vi "ELVIS III v1.0 Build MUX Configuration DIO.vi"(11 "DIO Channel List":T4) -> (1 "Configuration Bitmask Array":bool[][](array[boolean]), 2 "Configration Bitcode Array":bool[][](array[boolean]), 3 "Channel Reservation List":T1)   [LabVIEW 2021]
uses:
  <vilib>/myRIO/Common/Instrument Driver Framework/myRIO v1.0/DIO/typedefs/DIO Channels List.ctl
  <vilib>/myRIO/Common/Instrument Driver Framework/myRIO v1.0/DIO/typedefs/DIO Channels Enum.ctl
  <vilib>/myRIO/Common/Instrument Driver Framework/ELVIS III v1.0/Resource Manager/typedefs/ELVIS III v1.0 Channel Reservation List.ctl
  <vilib>/myRIO/Common/Instrument Driver Framework/ELVIS III v1.0/Resource Manager/typedefs/ELVIS III v1.0 Channel Reservation Info.ctl
  <vilib>/myRIO/Common/Instrument Driver Framework/ELVIS III v1.0/Resource Manager/typedefs/ELVIS III v1.0 Connector List.ctl
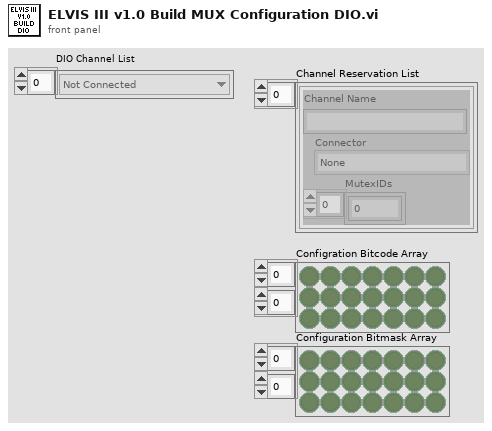
[diagram p1: front panel]
types:
  T1 = typedef "ELVIS III v1.0 Channel Reservation List.ctl" = T2[]
  T2 = typedef "ELVIS III v1.0 Channel Reservation Info.ctl" = cluster{"Channel Name":string, "Connector":T3, "MutexIDs":u32[]}
  T3 = typedef "ELVIS III v1.0 Connector List.ctl" = enum32{"None", "ConnectorA", "ConnectorB"}
  T4 = typedef "DIO Channels List.ctl" = T5[]
  T5 = typedef "DIO Channels Enum.ctl" = enum16{"Not Connected", "C/DIO0", "C/DIO1", "C/DIO2", "C/DIO3", "C/DIO4", "C/DIO5", "C/DIO6", "C/DIO7", "A/DIO0", "A/DIO1", "A/DIO2", "A/DIO3", "A/DIO4", "A/DIO5", "A/DIO6", "A/DIO7", "A/DIO8", "A/DIO9", "A/DIO10", "A/DIO11", "A/DIO12", "A/DIO13", "A/DIO14", "A/DIO15", "A/DIO16", "A/DIO17", "A/DIO18", "A/DIO19", "B/DIO0", "B/DIO1", "B/DIO2", "B/DIO3", "B/DIO4", "B/DIO5", "B/DIO6", "B/DIO7", "B/DIO8", "B/DIO9", "B/DIO10", "B/DIO11", "B/DIO12", "B/DIO13", "B/DIO14", "B/DIO15", "B/DIO16", "B/DIO17", "B/DIO18", "B/DIO19", "LED0", "LED1", "LED2", "LED3", "Button0", "DIO/DIO0", "DIO/DIO1", "DIO/DIO2", "DIO/DIO3", "DIO/DIO4", "DIO/DIO5", "DIO/DIO6", "DIO/DIO7", "DIO/DIO8", "DIO/DIO9", "SPI/CS0", "SPI/CS1", "SPI/CS2", "SPI/CS3", "LED RADIO (Green)", "LED RADIO (Red)", "LED COMM (Green)", "LED COMM (Red)", "LED MODE (Green)", "LED MODE (Red)"}
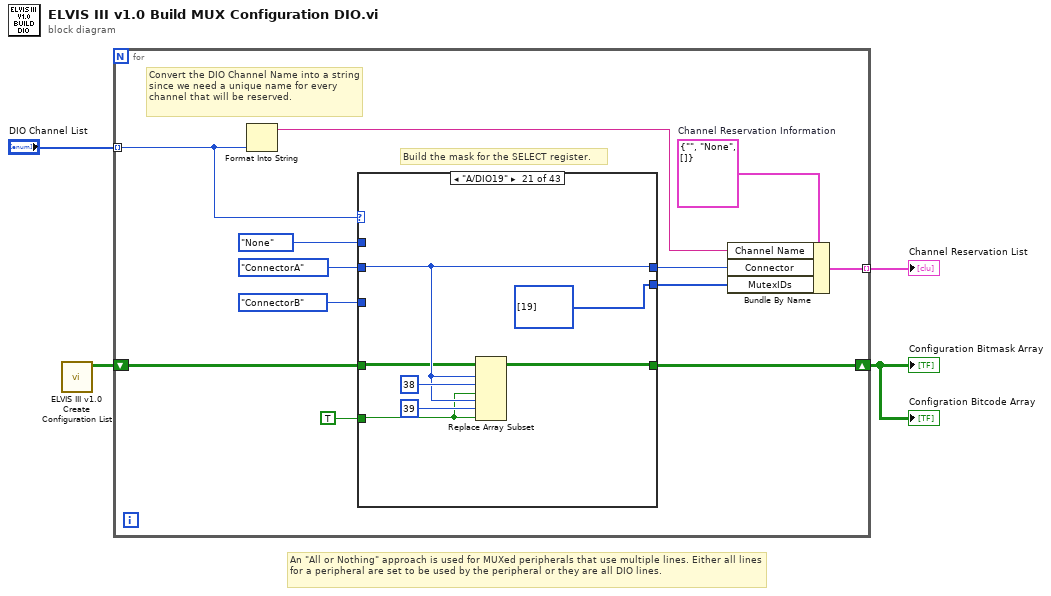
[diagram p0: block diagram]
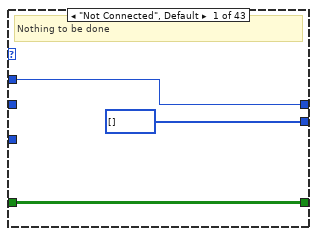
[diagram p2: hidden frame]
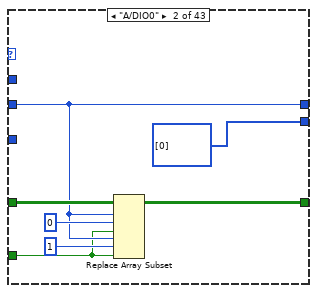
[diagram p3: hidden frame]
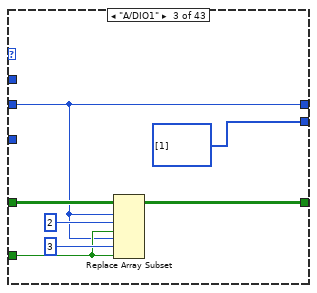
[diagram p4: hidden frame]
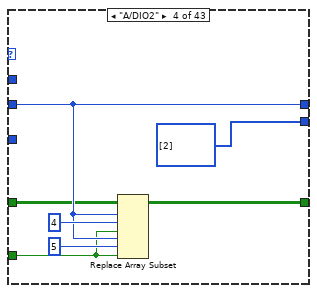
[diagram p5: hidden frame]
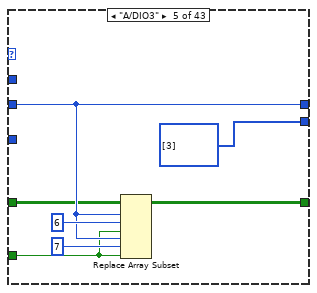
[diagram p6: hidden frame]
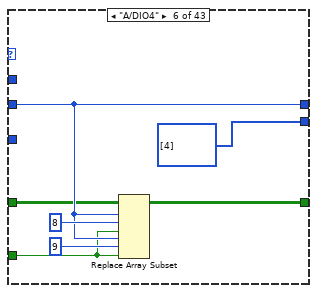
[diagram p7: hidden frame]
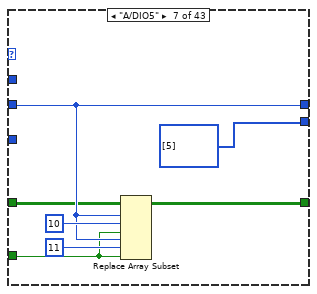
[diagram p8: hidden frame]
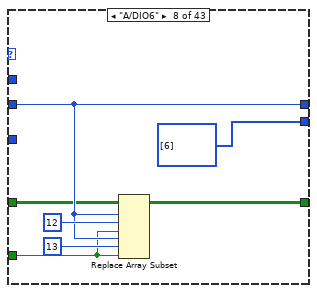
[diagram p9: hidden frame]
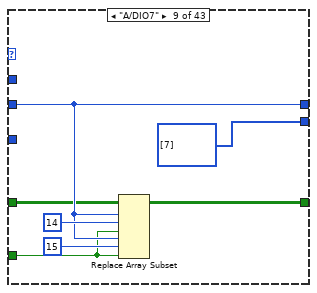
[diagram p10: hidden frame]
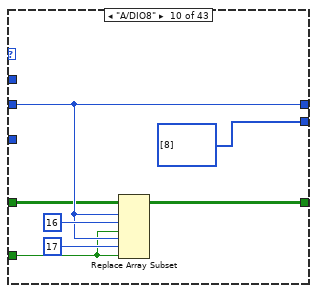
[diagram p11: hidden frame]
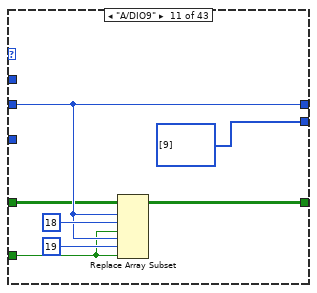
[diagram p12: hidden frame]
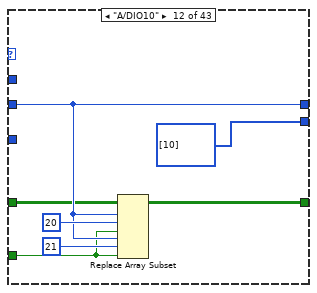
[diagram p13: hidden frame]
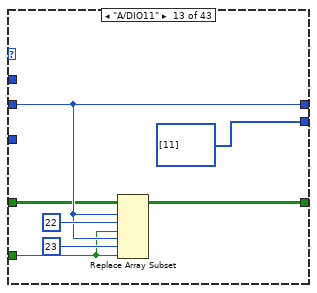
[diagram p14: hidden frame]
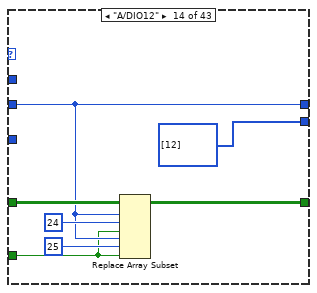
[diagram p15: hidden frame]
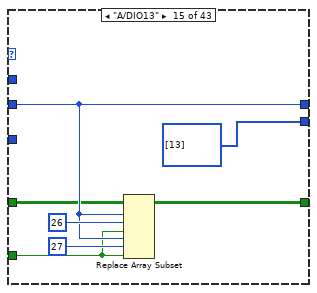
[diagram p16: hidden frame]
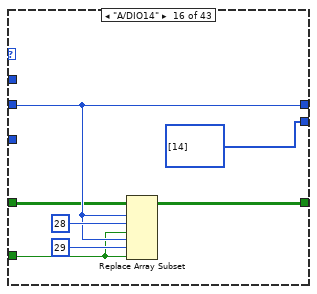
[diagram p17: hidden frame]
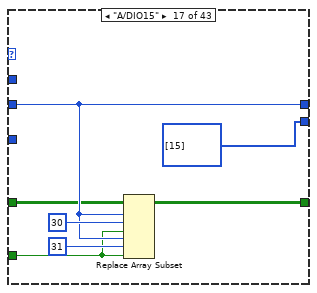
[diagram p18: hidden frame]
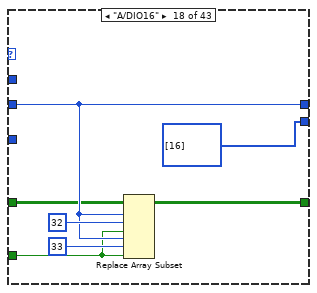
[diagram p19: hidden frame]
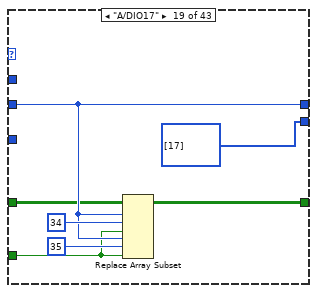
[diagram p20: hidden frame]
diagram:
  # "An \"All or Nothing\" approach is used for MUXed peripherals that use multiple lines. Either all lines for a peripheral are set to be used by the peripheral or they are all DIO lines."
  n1 = call <vilib>:"ELVIS III v1.0 Create Configuration List.vi"() -> ("Bitmask Array"=w4:bool[][])  [unwired: 11 in]
  n2 = for {
    shift-right: [w13] -> w1
    shift-left: w4 -> [w14]
    tunnel: "DIO Channel List" -> [w8] mode=indexing
    tunnel: [w9] -> w2 mode=indexing
    w12 = T2 {"Channel Name"="", "Connector"=enum."None", "MutexIDs"=[]}  # Channel Reservation Information
    # "Convert the DIO Channel Name into a string since we need a unique name for every channel that will be reserved."
    # "Build the mask for the SELECT register."
    n3 = Format Into String(w8) -> (resulting string=w7:string)  [unwired: 3 in, 1 out]
    n4 = case shown="\"A/DIO19\"" w8 {
      tunnel: w14 -> [w19 w25 w31 w35 w42 w50 w56 w63 w71 w78 w84 w92 w98 w108 w112 w119 w126 w134 w140 w148 w155 w164 w171 w178 w185 w192 w199 w206 w213 w218 w227 w232 w238 w246 w255 w260 w269 w273 w281 w288 w295 w300 w303]
      tunnel: [w19 w20 w29 w36 w43 w49 w57 w64 w70 w77 w85 w91 w99 w105 w113 w120 w127 w133 w141 w147 w154 w160 w169 w174 w181 w190 w197 w204 w209 w217 w225 w231 w239 w245 w253 w259 w267 w274 w282 w287 w294 w300 w303] -> w13
      tunnel: ELVIS_III_v1.0_Connector_List."None" ("Connector List") -> [w18 _ _ _ _ _ _ _ _ _ _ _ _ _ _ _ _ _ _ _ _ _ _ _ _ _ _ _ _ _ _ _ _ _ _ _ _ _ _ _ _ w301 w305]
      tunnel: TRUE ("new element/subarray") -> [_ w21 w30 w34 w41 w48 w55 w62 w69 w76 w83 w90 w97 w104 w111 w118 w125 w132 w139 w146 w153 w163 w170 w177 w184 w191 w198 w205 w212 w216 w226 w230 w237 w244 w254 w258 w268 w272 w279 w286 w293 _ _]
      tunnel: [u32[] [] ("MutexIDs") u32[] [0] u32[] [1] u32[] [2] u32[] [3] u32[] [4] u32[] [5] u32[] [6] u32[] [7] u32[] [8] u32[] [9] u32[] [10] u32[] [11] u32[] [12] u32[] [13] u32[] [14] u32[] [15] u32[] [16] u32[] [17] u32[] [18] u32[] [19] u32[] [0] u32[] [1] u32[] [2] u32[] [3] u32[] [4] u32[] [5] u32[] [6] u32[] [7] u32[] [8] u32[] [9] u32[] [10] u32[] [11] u32[] [12] u32[] [13] u32[] [14] u32[] [15] u32[] [16] u32[] [17] u32[] [18] u32[] [19] u32[] [] ("MutexIDs") u32[] [] ("MutexIDs")] -> w10
      tunnel: [w18 w23 w27 w38 w45 w52 w59 w66 w72 w79 w87 w94 w101 w107 w115 w122 w129 w136 w143 w150 w157 w162 w167 w176 w183 w188 w195 w202 w211 w220 w223 w234 w241 w248 w251 w262 w265 w276 w280 w290 w297 w301 w305] -> w11
      tunnel: ELVIS_III_v1.0_Connector_List."ConnectorA" ("Connector List") -> [_ w23 w27 w38 w45 w52 w59 w66 w72 w79 w87 w94 w101 w107 w115 w122 w129 w136 w143 w150 w157 _ _ _ _ _ _ _ _ _ _ _ _ _ _ _ _ _ _ _ _ _ _]
      tunnel: ELVIS_III_v1.0_Connector_List."ConnectorB" ("Connector List") -> [_ _ _ _ _ _ _ _ _ _ _ _ _ _ _ _ _ _ _ _ _ w162 w167 w176 w183 w188 w195 w202 w211 w220 w223 w234 w241 w248 w251 w262 w265 w276 w280 w290 w297 _ _]
      frame "Not Connected", Default {
        # "Nothing to be done"
      }
      frame "A/DIO0" {
        n5 = Replace Array Subset(array=w25, new element #1=w21, index (row) #1=w23, index (col) #1=0 ("disabled index (col)"), new element #2=w21, index (row) #2=w23, index (col) #2=1 ("disabled index (col)")) -> (w20:bool[][])
      }
      frame "A/DIO1" {
        n6 = Replace Array Subset(array=w31, new element #1=w30, index (row) #1=w27, index (col) #1=2 ("disabled index (col)"), new element #2=w30, index (row) #2=w27, index (col) #2=3 ("disabled index (col)")) -> (w29:bool[][])
      }
      frame "A/DIO2" {
        n7 = Replace Array Subset(array=w35, new element #1=w34, index (row) #1=w38, index (col) #1=4 ("disabled index (col)"), new element #2=w34, index (row) #2=w38, index (col) #2=5 ("disabled index (col)")) -> (w36:bool[][])
      }
      frame "A/DIO3" {
        n8 = Replace Array Subset(array=w42, new element #1=w41, index (row) #1=w45, index (col) #1=6 ("disabled index (col)"), new element #2=w41, index (row) #2=w45, index (col) #2=7 ("disabled index (col)")) -> (w43:bool[][])
      }
      frame "A/DIO4" {
        n9 = Replace Array Subset(array=w50, new element #1=w48, index (row) #1=w52, index (col) #1=8 ("disabled index (col)"), new element #2=w48, index (row) #2=w52, index (col) #2=9 ("disabled index (col)")) -> (w49:bool[][])
      }
      frame "A/DIO5" {
        n10 = Replace Array Subset(array=w56, new element #1=w55, index (row) #1=w59, index (col) #1=10 ("disabled index (col)"), new element #2=w55, index (row) #2=w59, index (col) #2=11 ("disabled index (col)")) -> (w57:bool[][])
      }
      frame "A/DIO6" {
        n11 = Replace Array Subset(array=w63, new element #1=w62, index (row) #1=w66, index (col) #1=12 ("disabled index (col)"), new element #2=w62, index (row) #2=w66, index (col) #2=13 ("disabled index (col)")) -> (w64:bool[][])
      }
      frame "A/DIO7" {
        n12 = Replace Array Subset(array=w71, new element #1=w69, index (row) #1=w72, index (col) #1=14 ("disabled index (col)"), new element #2=w69, index (row) #2=w72, index (col) #2=15 ("disabled index (col)")) -> (w70:bool[][])
      }
      frame "A/DIO8" {
        n13 = Replace Array Subset(array=w78, new element #1=w76, index (row) #1=w79, index (col) #1=16 ("disabled index (col)"), new element #2=w76, index (row) #2=w79, index (col) #2=17 ("disabled index (col)")) -> (w77:bool[][])
      }
      frame "A/DIO9" {
        n14 = Replace Array Subset(array=w84, new element #1=w83, index (row) #1=w87, index (col) #1=18 ("disabled index (col)"), new element #2=w83, index (row) #2=w87, index (col) #2=19 ("disabled index (col)")) -> (w85:bool[][])
      }
      frame "A/DIO10" {
        n15 = Replace Array Subset(array=w92, new element #1=w90, index (row) #1=w94, index (col) #1=20 ("disabled index (col)"), new element #2=w90, index (row) #2=w94, index (col) #2=21 ("disabled index (col)")) -> (w91:bool[][])
      }
      frame "A/DIO11" {
        n16 = Replace Array Subset(array=w98, new element #1=w97, index (row) #1=w101, index (col) #1=22 ("disabled index (col)"), new element #2=w97, index (row) #2=w101, index (col) #2=23 ("disabled index (col)")) -> (w99:bool[][])
      }
      frame "A/DIO12" {
        n17 = Replace Array Subset(array=w108, new element #1=w104, index (row) #1=w107, index (col) #1=24 ("disabled index (col)"), new element #2=w104, index (row) #2=w107, index (col) #2=25 ("disabled index (col)")) -> (w105:bool[][])
      }
      frame "A/DIO13" {
        n18 = Replace Array Subset(array=w112, new element #1=w111, index (row) #1=w115, index (col) #1=26 ("disabled index (col)"), new element #2=w111, index (row) #2=w115, index (col) #2=27 ("disabled index (col)")) -> (w113:bool[][])
      }
      frame "A/DIO14" {
        n19 = Replace Array Subset(array=w119, new element #1=w118, index (row) #1=w122, index (col) #1=28 ("disabled index (col)"), new element #2=w118, index (row) #2=w122, index (col) #2=29 ("disabled index (col)")) -> (w120:bool[][])
      }
      frame "A/DIO15" {
        n20 = Replace Array Subset(array=w126, new element #1=w125, index (row) #1=w129, index (col) #1=30 ("disabled index (col)"), new element #2=w125, index (row) #2=w129, index (col) #2=31 ("disabled index (col)")) -> (w127:bool[][])
      }
      frame "A/DIO16" {
        n21 = Replace Array Subset(array=w134, new element #1=w132, index (row) #1=w136, index (col) #1=32 ("disabled index (col)"), new element #2=w132, index (row) #2=w136, index (col) #2=33 ("disabled index (col)")) -> (w133:bool[][])
      }
      frame "A/DIO17" {
        n22 = Replace Array Subset(array=w140, new element #1=w139, index (row) #1=w143, index (col) #1=34 ("disabled index (col)"), new element #2=w139, index (row) #2=w143, index (col) #2=35 ("disabled index (col)")) -> (w141:bool[][])
      }
      frame "A/DIO18" {
        n23 = Replace Array Subset(array=w148, new element #1=w146, index (row) #1=w150, index (col) #1=36 ("disabled index (col)"), new element #2=w146, index (row) #2=w150, index (col) #2=37 ("disabled index (col)")) -> (w147:bool[][])
      }
      frame "A/DIO19" {
        n24 = Replace Array Subset(array=w155, new element #1=w153, index (row) #1=w157, index (col) #1=38 ("disabled index (col)"), new element #2=w153, index (row) #2=w157, index (col) #2=39 ("disabled index (col)")) -> (w154:bool[][])
      }
      frame "B/DIO0" {
        n25 = Replace Array Subset(array=w164, new element #1=w163, index (row) #1=w162, index (col) #1=0 ("disabled index (col)"), new element #2=w163, index (row) #2=w162, index (col) #2=1 ("disabled index (col)")) -> (w160:bool[][])
      }
      frame "B/DIO1" {
        n26 = Replace Array Subset(array=w171, new element #1=w170, index (row) #1=w167, index (col) #1=2 ("disabled index (col)"), new element #2=w170, index (row) #2=w167, index (col) #2=3 ("disabled index (col)")) -> (w169:bool[][])
      }
      frame "B/DIO2" {
        n27 = Replace Array Subset(array=w178, new element #1=w177, index (row) #1=w176, index (col) #1=4 ("disabled index (col)"), new element #2=w177, index (row) #2=w176, index (col) #2=5 ("disabled index (col)")) -> (w174:bool[][])
      }
      frame "B/DIO3" {
        n28 = Replace Array Subset(array=w185, new element #1=w184, index (row) #1=w183, index (col) #1=6 ("disabled index (col)"), new element #2=w184, index (row) #2=w183, index (col) #2=7 ("disabled index (col)")) -> (w181:bool[][])
      }
      frame "B/DIO4" {
        n29 = Replace Array Subset(array=w192, new element #1=w191, index (row) #1=w188, index (col) #1=8 ("disabled index (col)"), new element #2=w191, index (row) #2=w188, index (col) #2=9 ("disabled index (col)")) -> (w190:bool[][])
      }
      frame "B/DIO5" {
        n30 = Replace Array Subset(array=w199, new element #1=w198, index (row) #1=w195, index (col) #1=10 ("disabled index (col)"), new element #2=w198, index (row) #2=w195, index (col) #2=11 ("disabled index (col)")) -> (w197:bool[][])
      }
      frame "B/DIO6" {
        n31 = Replace Array Subset(array=w206, new element #1=w205, index (row) #1=w202, index (col) #1=12 ("disabled index (col)"), new element #2=w205, index (row) #2=w202, index (col) #2=13 ("disabled index (col)")) -> (w204:bool[][])
      }
      frame "B/DIO7" {
        n32 = Replace Array Subset(array=w213, new element #1=w212, index (row) #1=w211, index (col) #1=14 ("disabled index (col)"), new element #2=w212, index (row) #2=w211, index (col) #2=15 ("disabled index (col)")) -> (w209:bool[][])
      }
      frame "B/DIO8" {
        n33 = Replace Array Subset(array=w218, new element #1=w216, index (row) #1=w220, index (col) #1=16 ("disabled index (col)"), new element #2=w216, index (row) #2=w220, index (col) #2=17 ("disabled index (col)")) -> (w217:bool[][])
      }
      frame "B/DIO9" {
        n34 = Replace Array Subset(array=w227, new element #1=w226, index (row) #1=w223, index (col) #1=18 ("disabled index (col)"), new element #2=w226, index (row) #2=w223, index (col) #2=19 ("disabled index (col)")) -> (w225:bool[][])
      }
      frame "B/DIO10" {
        n35 = Replace Array Subset(array=w232, new element #1=w230, index (row) #1=w234, index (col) #1=20 ("disabled index (col)"), new element #2=w230, index (row) #2=w234, index (col) #2=21 ("disabled index (col)")) -> (w231:bool[][])
      }
      frame "B/DIO11" {
        n36 = Replace Array Subset(array=w238, new element #1=w237, index (row) #1=w241, index (col) #1=22 ("disabled index (col)"), new element #2=w237, index (row) #2=w241, index (col) #2=23 ("disabled index (col)")) -> (w239:bool[][])
      }
      frame "B/DIO12" {
        n37 = Replace Array Subset(array=w246, new element #1=w244, index (row) #1=w248, index (col) #1=24 ("disabled index (col)"), new element #2=w244, index (row) #2=w248, index (col) #2=25 ("disabled index (col)")) -> (w245:bool[][])
      }
      frame "B/DIO13" {
        n38 = Replace Array Subset(array=w255, new element #1=w254, index (row) #1=w251, index (col) #1=26 ("disabled index (col)"), new element #2=w254, index (row) #2=w251, index (col) #2=27 ("disabled index (col)")) -> (w253:bool[][])
      }
      frame "B/DIO14" {
        n39 = Replace Array Subset(array=w260, new element #1=w258, index (row) #1=w262, index (col) #1=28 ("disabled index (col)"), new element #2=w258, index (row) #2=w262, index (col) #2=29 ("disabled index (col)")) -> (w259:bool[][])
      }
      frame "B/DIO15" {
        n40 = Replace Array Subset(array=w269, new element #1=w268, index (row) #1=w265, index (col) #1=30 ("disabled index (col)"), new element #2=w268, index (row) #2=w265, index (col) #2=31 ("disabled index (col)")) -> (w267:bool[][])
      }
      frame "B/DIO16" {
        n41 = Replace Array Subset(array=w273, new element #1=w272, index (row) #1=w276, index (col) #1=32 ("disabled index (col)"), new element #2=w272, index (row) #2=w276, index (col) #2=33 ("disabled index (col)")) -> (w274:bool[][])
      }
      frame "B/DIO17" {
        n42 = Replace Array Subset(array=w281, new element #1=w279, index (row) #1=w280, index (col) #1=34 ("disabled index (col)"), new element #2=w279, index (row) #2=w280, index (col) #2=35 ("disabled index (col)")) -> (w282:bool[][])
      }
      frame "B/DIO18" {
        n43 = Replace Array Subset(array=w288, new element #1=w286, index (row) #1=w290, index (col) #1=36 ("disabled index (col)"), new element #2=w286, index (row) #2=w290, index (col) #2=37 ("disabled index (col)")) -> (w287:bool[][])
      }
      frame "B/DIO19" {
        n44 = Replace Array Subset(array=w295, new element #1=w293, index (row) #1=w297, index (col) #1=38 ("disabled index (col)"), new element #2=w293, index (row) #2=w297, index (col) #2=39 ("disabled index (col)")) -> (w294:bool[][])
      }
      frame "LED0".."LED3" {
      }
      frame "Button0" {
      }
    }
    n45 = Bundle By Name(cluster=w12, "Channel Name"=w7, "Connector"=w11, "MutexIDs"=w10) -> (w9:T2)
  }
  "Configuration Bitmask Array" <- w1
  "Channel Reservation List" <- w2
  "Configration Bitcode Array" <- w1
